vi "Raster_2DOutput_wCounter_82_EXP Two counters.vi"(2 "Save File path":path, 3 "Save?":bool=TRUE, 6 "error in":errorcluster, 7 "Update Rate (Hz)":dbl=100.0, 8 "Y Parameters":T1={"Number of Y Steps"=200, "Max Y (V)"=2.0, "Min Y (V)"=-2.0}, 9 "X Parameters":T2={"Number of X Steps"=200, "Max X (V)"=2.0, "Min X (V)"=-2.0}) -> (0 "error out":errorcluster, 1 "Intensity Graph":dbl[][](graph))   [LabVIEW 2012]
uses:
  <vilib>/DAQmx/write.llb/DAQmx Write (Analog 2D DBL NChan NSamp).vi
  <vilib>/DAQmx/read.llb/DAQmx Read (Counter 1D U32 1Chan NSamp).vi
  <vilib>/DAQmx/create/channels.llb/DAQmx Create Channel (CI-Count Edges).vi
  <vilib>/DAQmx/configure/timing.llb/DAQmx Timing (Sample Clock).vi
  <vilib>/DAQmx/create/channels.llb/DAQmx Create Channel (AO-Voltage-Basic).vi
  <vilib>/DAQmx/miscellaneous.llb/DAQmx Fill In Error Info.vi
  <resource>/objmgr/daqmx.rc
panel:
  out "TotalSampPerChanAcquired":dbl
  in  "stop":bool
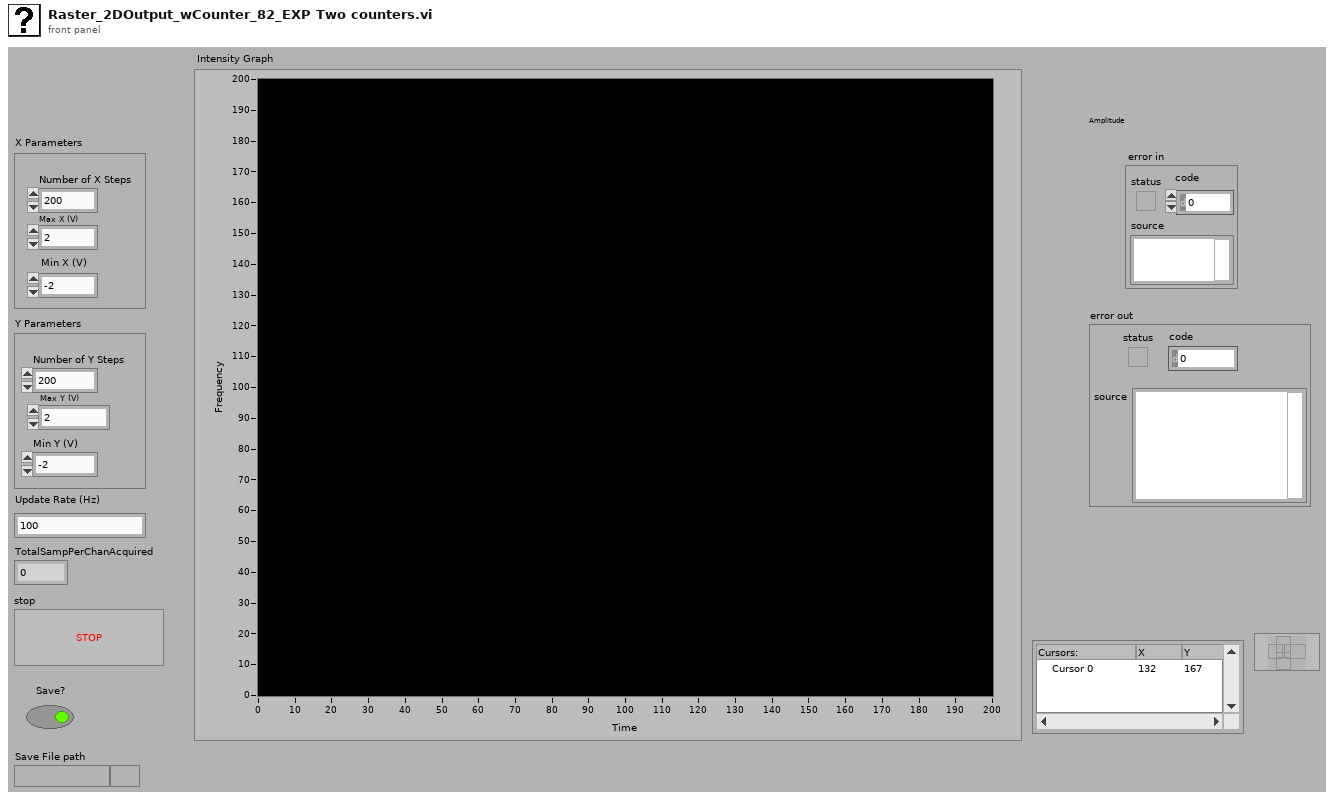
[diagram p1: front panel]
types:
  T1 = cluster{"Number of Y Steps":i32, "Max Y (V)":dbl, "Min Y (V)":dbl}
  T2 = cluster{"Number of X Steps":i32, "Max X (V)":dbl, "Min X (V)":dbl}
  T3 = typedef "imagedata.ctl" = cluster{"image type":i32, "image depth":i32, "image":u8[], "mask":u8[], "colors":u32[], "Rectangle":cluster{"left":i16, "top":i16, "right":i16, "bottom":i16}}
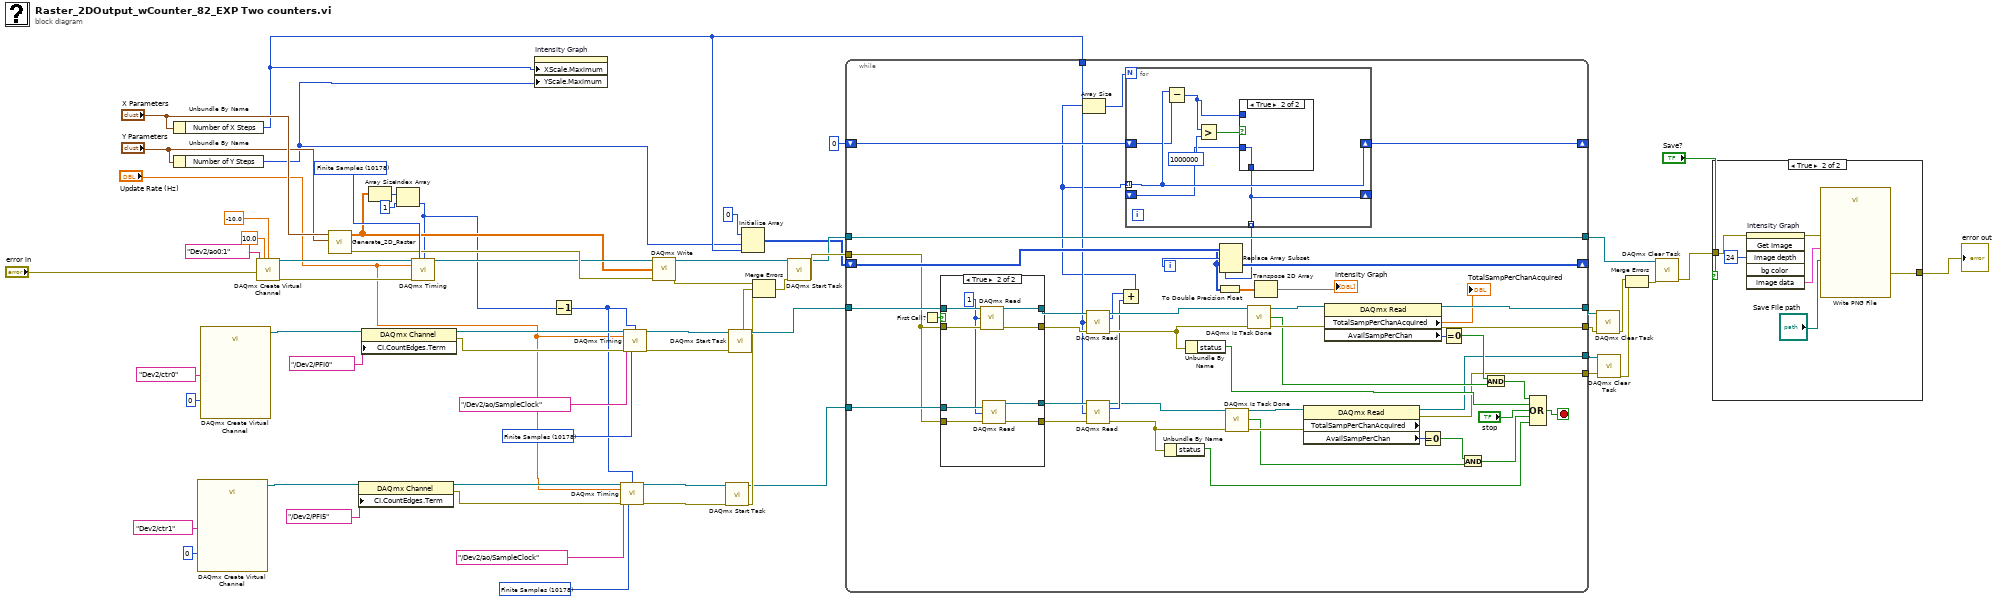
[diagram p0: block diagram]
diagram:
  w20 = 10178 items=["Finite Samples"=10178, "Continuous Samples"=10123, "Hardware Timed Single Point"=12522] ("sample mode")
  w53 = 10178 items=["Finite Samples"=10178, "Continuous Samples"=10123, "Hardware Timed Single Point"=12522] ("sample mode")
  w54 = 10178 items=["Finite Samples"=10178, "Continuous Samples"=10123, "Hardware Timed Single Point"=12522] ("sample mode")
  n1 = Unbundle By Name("X Parameters") -> ("Number of X Steps"=w24:i32)
  n2 = Unbundle By Name("Y Parameters") -> ("Number of Y Steps"=w23:i32)
  n3 = call-poly <vilib>:"DAQmx Create Virtual Channel.vi"("initial count"=u32 0, "counter"=tag "Dev2/ctr1") -> ("task out"=w18:refnum<k21>)  [unwired: 6 in, 7 out]
  n4 = call-poly <vilib>:"DAQmx Create Virtual Channel.vi"("initial count"=u32 0, "counter"=tag "Dev2/ctr0") -> ("task out"=w32:refnum<k21>)  [unwired: 6 in, 7 out]
  n5 = call-poly <vilib>:"DAQmx Create Virtual Channel.vi"("maximum value"=10.0, "minimum value"=-10.0, "physical channels"=tag "Dev2/ao0:1", "error in"="error in") -> ("task out"=w62:refnum<k21>, "error out"=w61:errorcluster)  [unwired: 5 in, 5 out]
  n6 = call "Generate_2D_Raster.vi"("Y Parameters"="Y Parameters", "X Parameters"="X Parameters") -> ("error IO"=w47:errorcluster, "Array"=w41:dbl[][])  [unwired: 1 in, 7 out]
  n7 = property class="DAQmx Channel"(reference=w18, "CI.CountEdges.Term"=tag "/Dev2/PFI5") -> (reference out=w17:refnum<k21>, error out=w16:errorcluster)  [unwired: 1 in]
  n8 = property class="DAQmx Channel"(reference=w32, "CI.CountEdges.Term"=tag "/Dev2/PFI0") -> (reference out=w31:refnum<k21>, error out=w30:errorcluster)  [unwired: 1 in]
  n9 = Array Size(array=w41) -> (size(s)=w40:i32[])
  n10 = Index Array(array=w40, index=1) -> (element=w11:i32)
  n11 = call-poly <vilib>:"DAQmx Timing.vi"("task/channels in"=w62, "sample mode"=w54, "samples per channel"=w11, "rate"="Update Rate (Hz)", "error in"=w61) -> ("task out"=w42:refnum<k21>)  [unwired: 2 in, 8 out]
  n12 = property on="Intensity Graph" class="IntGraph (strict)"("XScale.Maximum"=w24, "YScale.Maximum"=w23) -> ()  [unwired: 2 in, 2 out]
  n13 = Decrement(x=w11) -> (x-1=w10:i32)
  n14 = call-poly <vilib>:"DAQmx Timing.vi"("task/channels in"=w17, "sample mode"=w20, "samples per channel"=w10, "rate"="Update Rate (Hz)", "source"=tag "/Dev2/ao/SampleClock", "error in"=w16) -> ("task out"=w21:refnum<k21>, "error out"=w13:errorcluster)  [unwired: 1 in, 7 out]
  n15 = call-poly <vilib>:"DAQmx Timing.vi"("task/channels in"=w31, "sample mode"=w53, "samples per channel"=w10, "rate"="Update Rate (Hz)", "source"=tag "/Dev2/ao/SampleClock", "error in"=w30) -> ("task out"=w59:refnum<k21>, "error out"=w25:errorcluster)  [unwired: 1 in, 7 out]
  n16 = call-poly <vilib>:"DAQmx Write.vi"("task/channels in"=w42, "data"=w41, "error in"=w47) -> ("task out"=w58:refnum<k21>, "error out"=w48:errorcluster)  [unwired: 1 in, 10 out]
  n17 = call <vilib>:"DAQmx Start Task.vi"("task/channels in"=w21, "error in"=w13) -> ("task out"=w6:refnum<k21>, "error out"=w7:errorcluster)  [unwired: 12 out]
  n18 = call <vilib>:"DAQmx Start Task.vi"("task/channels in"=w59, "error in"=w25) -> ("task out"=w55:refnum<k21>, "error out"=w8:errorcluster)  [unwired: 12 out]
  n19 = Initialize Array(u32 0, w23, w24) -> (w43:u32[][])
  n20 = Merge Errors(w48, w8, w7) -> (w49:errorcluster)
  n21 = call <vilib>:"DAQmx Start Task.vi"("task/channels in"=w58, "error in"=w49) -> ("task out"=w56:refnum<k21>, "error out"=w57:errorcluster)  [unwired: 12 out]
  n22 = while {
    tunnel: w56 -> [w101]
    tunnel: w57 -> [w80]
    tunnel: w55 -> [w108]
    tunnel: [w101] -> w52
    tunnel: w24 -> [w77]
    shift-right: [w102] -> _
    shift-left: w43 -> [w104]
    tunnel: [w97] -> w38
    tunnel: [w98] -> w37
    shift-right: [w84] -> _
    shift-left: u32 0 ("Numeric") -> [w83]
    tunnel: w6 -> [w81]
    tunnel: [w64] -> w5
    tunnel: [w63] -> w4
    i -> [w103]
    stop <- w109 stop-if-true
    n23 = First Call?() -> (First Call?: T/F=w105:bool)
    n24 = case shown="True" w105 {
      tunnel: w108 -> [w122 w131]
      tunnel: [w122 w130] -> w107
      tunnel: [w121 w129] -> w106
      tunnel: w80 -> [w121 w128]
      tunnel: w81 -> [w120 w127]
      tunnel: w80 -> [w119 w126]
      tunnel: [w120 w125] -> w79
      tunnel: [w119 w124] -> w78
      frame False {
      }
      frame True {
        w123 = 1 ("number of samples per channel")
        n25 = call-poly <vilib>:"DAQmx Read.vi"("task/channels in"=w131, "number of samples per channel"=w123, "error in"=w128) -> ("task out"=w130:refnum<k21>, "error out"=w129:errorcluster)  [unwired: 11 out]
        n26 = call-poly <vilib>:"DAQmx Read.vi"("task/channels in"=w127, "number of samples per channel"=w123, "error in"=w126) -> ("task out"=w125:refnum<k21>, "error out"=w124:errorcluster)  [unwired: 11 out]
      }
    }
    n27 = call-poly <vilib>:"DAQmx Read.vi"("task/channels in"=w107, "number of samples per channel"=w77, "error in"=w106) -> ("task out"=w99:refnum<k21>, "data"=w75:u32[], "error out"=w90:errorcluster)  [unwired: 1 in, 9 out]
    n28 = call-poly <vilib>:"DAQmx Read.vi"("task/channels in"=w79, "number of samples per channel"=w77, "error in"=w78) -> ("task out"=w70:refnum<k21>, "data"=w76:u32[], "error out"=w69:errorcluster)  [unwired: 1 in, 9 out]
    n29 = Add(x=w75, y=w76) -> (x+y=w74:u32[])
    n30 = Array Size(array=w74) -> (size(s)=w86:i32)
    n31 = for {
      N: w86 -> [_]
      tunnel: w74 -> [w116] mode=indexing
      shift-right: [w116] -> w84
      shift-left: w83 -> [w115]
      tunnel: [w111] -> w85 mode=indexing
      shift-right: [w111] -> _
      shift-left: _ -> [w110]
      n32 = Subtract(x=w116, y=w115) -> (x-y=w112:u32)
      n33 = Greater?(x=w112, y=u32 1000000) -> (0:w113:bool)
      n34 = case shown="True" w113 {
        tunnel: w112 -> [w117 _]
        tunnel: [w117 w118] -> w111
        tunnel: w110 -> [_ w118]
        frame False {
        }
        frame True {
        }
      }
    }
    n35 = Unbundle By Name(w69) -> ("status"=w65:bool)
    n36 = Unbundle By Name(w90) -> ("status"=w88:bool)
    n37 = Replace Array Subset(array=w104, new element=w85, index (row)=w103) -> (w102:u32[][])  [unwired: 1 in]
    n38 = To Double Precision Float(number=w102) -> (double precision float=w100:dbl[][])
    n39 = call <vilib>:"DAQmx Is Task Done.vi"("task/channels in"=w70, "error in"=w69) -> ("task out"=w73:refnum<k21>, "task done?"=w67:bool, "error out"=w72:errorcluster)  [unwired: 11 out]
    n40 = call <vilib>:"DAQmx Is Task Done.vi"("task/channels in"=w99, "error in"=w90) -> ("task out"=w96:refnum<k21>, "task done?"=w93:bool, "error out"=w95:errorcluster)  [unwired: 11 out]
    n41 = Transpose 2D Array(2D array=w100) -> (transposed array=→"Intensity Graph":dbl[][])
    n42 = property class="DAQmx Read" props=["TotalSampPerChanAcquired", "AvailSampPerChan"](reference=w73, error in=w72) -> (reference out=w64:refnum<k21>, error out=w63:errorcluster, "AvailSampPerChan"=w71:u32)  [unwired: 1 out]
    n43 = property class="DAQmx Read"(reference=w96, error in=w95) -> (reference out=w98:refnum<k21>, error out=w97:errorcluster, "TotalSampPerChanAcquired"=→"TotalSampPerChanAcquired":dbl, "AvailSampPerChan"=w92:u32)
    n44 = Equal To 0?(x=w71) -> (x = 0?=w68:bool)
    n45 = Equal To 0?(x=w92) -> (x = 0?=w91:bool)
    n46 = And(x=w68, y=w67) -> (x .and. y?=w66:bool)
    n47 = And(x=w91, y=w93) -> (x .and. y?=w87:bool)
    n48 = Compound Arithmetic op=OR(w87, w88, "stop", w66, w65) -> (w109:bool)
  }
  n49 = call <vilib>:"DAQmx Clear Task.vi"("task in"=w37, "error in"=w38) -> ("error out"=w1:errorcluster)  [unwired: 13 out]
  n50 = call <vilib>:"DAQmx Clear Task.vi"("task in"=w5, "error in"=w4) -> ("error out"=w2:errorcluster)  [unwired: 13 out]
  n51 = Merge Errors(w1, w2) -> (w3:errorcluster)
  n52 = call <vilib>:"DAQmx Clear Task.vi"("task in"=w52, "error in"=w3) -> ("error out"=w36:errorcluster)  [unwired: 13 out]
  n53 = case shown="True" "Save?" {
    tunnel: w36 -> [w132 w136]
    tunnel: [w132 w138] -> w35
    frame False {
    }
    frame True {
      n54 = invoke on="Intensity Graph" class="IntGraph (strict)" method="Get Image"(error in=w136, "image depth"=24 ("Image Depth")) -> (error out=w135:errorcluster, "image data"=w134:T3)  [unwired: 4 in, 4 out]
      n55 = call <vilib>:"Write PNG File.vi"("error in (no error)"=w135, "image data"=w134, "path to PNG file"="Save File path") -> ("error out"=w138:errorcluster)  [unwired: 7 in, 1 out]
    }
  }
  "error out" <- w35
